vi "Sleep.vi"(8 "error in (no error)":errorcluster, 11 "ISleepable in":refnum<class "ISleepable.lvclass">) -> (0 "error out":errorcluster, 3 "ISleepable out":refnum<class "ISleepable.lvclass">)   [LabVIEW 2009, in "ISleepable.lvclass"]
doc: "Puts the object into sleep mode."
uses:
  ISleepable.lvclass
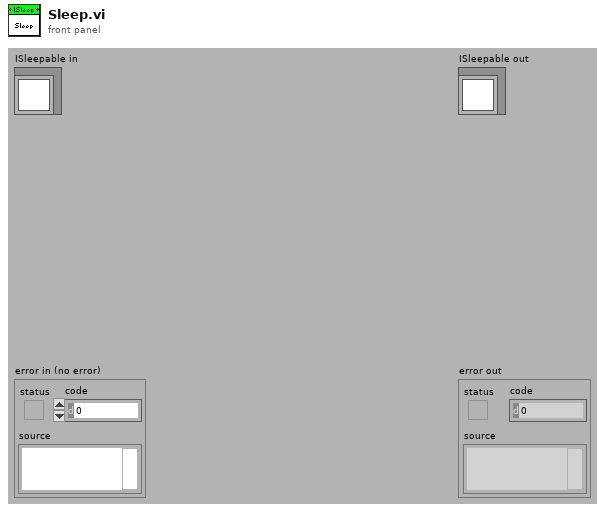
[diagram p1: front panel]
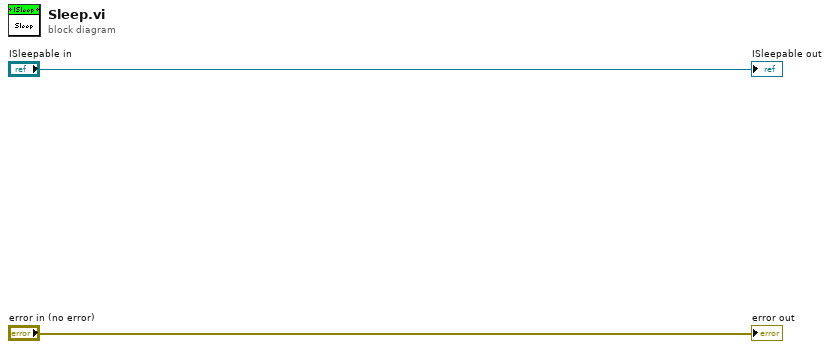
[diagram p0: block diagram]
diagram:
  "error out" <- "error in (no error)"
  "ISleepable out" <- "ISleepable in"
